vi "IAStateToCommand.vi"(10 "k":dbl=1.0 format="%#_13g", 11 "our_robots":T1[](array[typedef])) -> (3 "Message":T6 {"Vel Esquerda 3" format="%1_6f"; "Vel Esquerda 2" format="%1_6f"; "Vel Esquerda 1" format="%1_6f"; "Vel Direita 3" format="%1_6f"; "Vel Direita 2" format="%1_6f"; "Vel Direita 1" format="%1_6f"})   [LabVIEW 2017]
uses:
  grSim/Viewer Robot Command.ctl
  Core/AI Robot.ctl
  Intel/Functions Enum.ctl
  Intel/AttackerStates.ctl
  Path Planning/RRT/PathDests.ctl
  Path Planning/RRT/PathDest.ctl
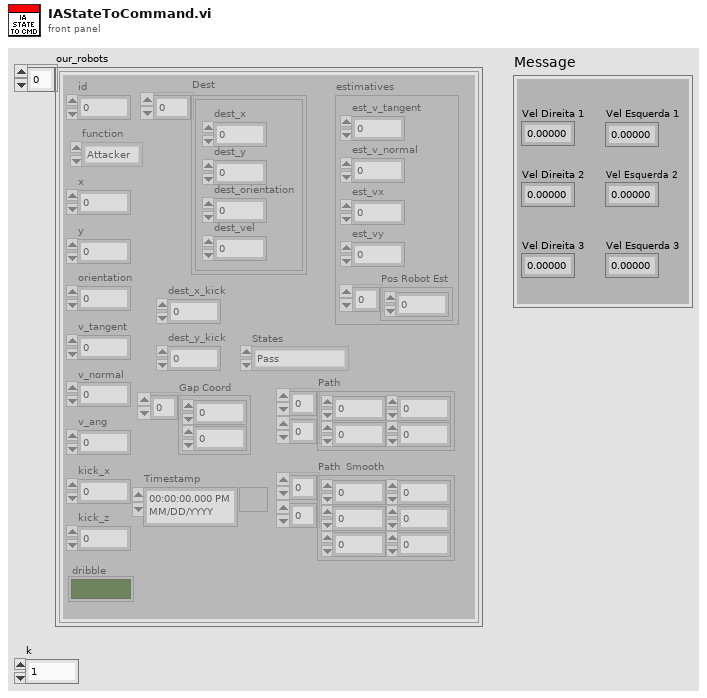
[diagram p1: front panel]
types:
  T1 = typedef "AI Robot.ctl" = cluster{"id":u32, "function":T2, "x":dbl, "y":dbl, "orientation":dbl, "v_tangent":dbl, "v_normal":dbl, "v_ang":dbl, "kick_x":dbl, "kick_z":dbl, "dribble":bool, "Timestamp":timestamp, "estimatives":cluster{"est_v_tangent":dbl, "est_v_normal":dbl, "est_vx":dbl, "est_vy":dbl, "Pos Robot Est":dbl[]}, "dest_x_kick":dbl, "dest_y_kick":dbl, "Gap Coord":dbl[], "States":T3, "Path ":dbl[][], "Path  Smooth":dbl[][], "Dest":T4}
  T2 = typedef "Functions Enum.ctl" = enum16{"Attacker", "Goalie", "Defender", "Striker", "Goto 0", "Dummy", "Kicker", "ZigZag"}
  T3 = typedef "AttackerStates.ctl" = enum16{"Pass", "GoToTangent", "BallGetting", "GoToKick", ""}
  T4 = typedef "PathDests.ctl" = T5[]
  T5 = typedef "PathDest.ctl" = cluster{"dest_x":dbl, "dest_y":dbl, "dest_orientation":dbl, "dest_vel":dbl}
  T6 = typedef "Viewer Robot Command.ctl" = cluster{"Vel Direita 1\n":dbl, "Vel Direita 2":dbl, "Vel Direita 3":dbl, "Vel Esquerda 1\n":dbl, "Vel Esquerda 2":dbl, "Vel Esquerda 3":dbl}
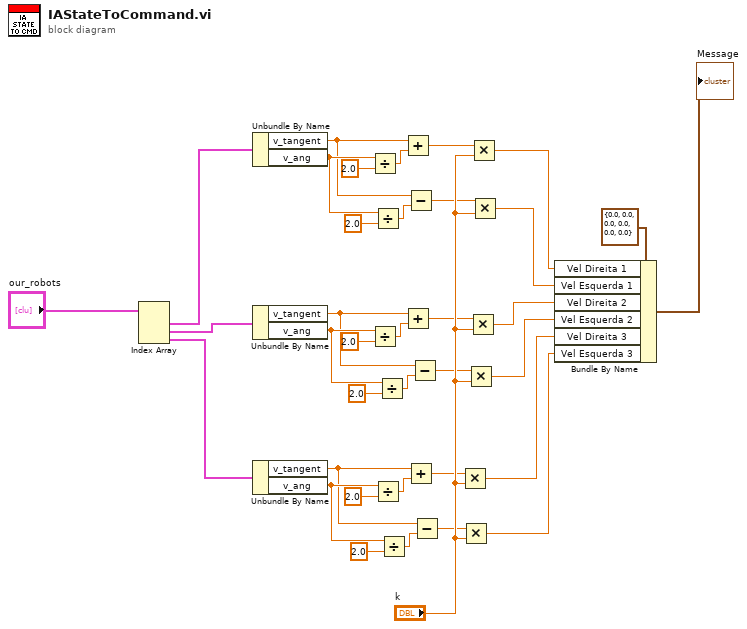
[diagram p0: block diagram]
diagram:
  n1 = Index Array(array="our_robots") -> (element #1=w35:T1, element #2=w37:T1, element #3=w36:T1)  [unwired: 3 in]
  n2 = Unbundle By Name(w35) -> ("v_tangent"=w12:dbl, "v_ang"=w13:dbl)
  n3 = Unbundle By Name(w37) -> ("v_tangent"=w16:dbl, "v_ang"=w17:dbl)
  n4 = Unbundle By Name(w36) -> ("v_tangent"=w20:dbl, "v_ang"=w21:dbl)
  n5 = Divide(x=w13, y=2.0) -> (x/y=w3:dbl)
  n6 = Divide(x=w17, y=2.0) -> (x/y=w6:dbl)
  n7 = Divide(x=w13, y=2.0) -> (x/y=w11:dbl)
  n8 = Divide(x=w21, y=2.0) -> (x/y=w7:dbl)
  n9 = Divide(x=w17, y=2.0) -> (x/y=w14:dbl)
  n10 = Divide(x=w21, y=2.0) -> (x/y=w19:dbl)
  n11 = Add(x=w12, y=w3) -> (x+y=w9:dbl)
  n12 = Add(x=w16, y=w6) -> (x+y=w23:dbl)
  n13 = Subtract(x=w12, y=w11) -> (x-y=w22:dbl)
  n14 = Add(x=w20, y=w7) -> (x+y=w25:dbl)
  n15 = Subtract(x=w16, y=w14) -> (x-y=w24:dbl)
  n16 = Subtract(x=w20, y=w19) -> (x-y=w26:dbl)
  n17 = Multiply(x=w25, y="k") -> (x*y=w32:dbl)
  n18 = Multiply(x=w26, y="k") -> (x*y=w33:dbl)
  n19 = Multiply(x=w24, y="k") -> (x*y=w31:dbl)
  n20 = Multiply(x=w23, y="k") -> (x*y=w30:dbl)
  n21 = Multiply(x=w9, y="k") -> (x*y=w28:dbl)
  n22 = Multiply(x=w22, y="k") -> (x*y=w29:dbl)
  n23 = Bundle By Name(cluster=T6 {"Vel Direita 1\n"=0.0, "Vel Direita 2"=0.0, "Vel Direita 3"=0.0, "Vel Esquerda 1\n"=0.0, "Vel Esquerda 2"=0.0, "Vel Esquerda 3"=0.0} ("Message"), "Vel Direita 1"=w28, "Vel Esquerda 1"=w29, "Vel Direita 2"=w30, "Vel Esquerda 2"=w31, "Vel Direita 3"=w32, "Vel Esquerda 3"=w33) -> (→"Message":T6)
